vi "AprilTag Target Package Code 1.vi"(0 "Camera List":string[](array[string]), 1 "Instance":i32) -> ()   [LabVIEW 2025]
uses:
  Camera Set Up/Ctrl/White Balance.ctl
  Camera Info.ctl
  State Machine/AprialTag States.ctl
  State Machine/AprialTag Main Cluster.ctl
  <vilib>/vision/Image Controls.llb/IMAQ Image.ctl
  Steam Type.ctl
  Camera Set Up/Event/Event Setup Types.ctl
  <vilib>/Utility/config.llb/Read Key (String).vi
  <vilib>/Utility/config.llb/Write Key (String).vi
  <vilib>/Utility/config.llb/NI_LVConfig.lvlib
  <vilib>/ptbypt/NI_PtbyPt.lvlib
panel:
  in  "Main":T1(tab)
  out "Running":bool
  out "Image":T2(plugin-control)
  out "Camera Name":string="cam0"
  in  "Settings":bool
  out "FPS":dbl format="%#.0f"
  out "Height":i32=360
  out "Width":i32=640
  out "Target Info":dbl[][](array[numeric]) format="%.1f"
  in  "Camera Setting":bool
  in  "Home":bool
  in  "Robot Calibration Cluster":T3={"Camera FOV Vert View Angle (deg)"=75.0, "Camera FOV Hor View Angle (deg)"=90.0, "Distance Correction Factor"=3.952} {"Distance Correction Factor" format="%#_13g"; "Camera FOV Hor View Angle (deg)" format="%#_13g"; "Camera FOV Vert View Angle (deg)" format="%#_13g"}
  in  "decimate":dbl=4.0 format="%#_13g"
  out "Camera Name 2":string="cam0"
  in  "Save":bool
  in  "Timeout":u32
  out "Distance (tag-size units)":dbl
  in  "Gamma":i32(slide)=50 min=0 max=100 scale=0.0..100.0
  in  "Brightness":i32(slide)=50 min=0 max=100 scale=0.0..100.0
  in  "Exposure":dbl(slide)=2.0 min=0.0 max=100.0 step=0.01 scale=0.0..100.0
  in  "Gain":i32(slide)=50 min=0 max=100 scale=0.0..100.0
  in  "Contrast":i32(slide)=50 min=0 max=100 scale=0.0..100.0
  in  "Sharpness":i32(slide)=50 min=0 max=100 scale=0.0..100.0
  in  "VideoMode":u16(ring)=20 items=["640x480 MJPG 60.00fps", "640x480 YUY2 60.00fps", "1280x720 MJPG 60.00fps", "1280x720 YUY2 60.00fps", "1600x1304 MJPG 60.00fps", "1600x1304 YUY2 60.00fps"]
  in  "White Balance":T4=enum."Hold current"
  out "Camera Image":T2(plugin-control)
  in  "Hue":i32(slide)=50 min=0 max=100 scale=0.0..100.0
  in  "Saturation":i32(slide)=50 min=0 max=100 scale=0.0..100.0
  out "Camera Name 3":string="cam0"
  in  "Reset Camera":bool
  in  "Camera Save Settings":bool caption="Save"
  out "Width 2":i32=640 caption="Width"
  out "Height 2":i32=360 caption="Height"
  in  "Home 2":bool caption="Home"
  # "Distance"
  # "Angle"
  # "Tag #"
  # "Yaw"
  # "Pitch"
  # "Roll"
  # "Distance Correction Factor:\nCalibration for the camera. Take three measurements at 24\", 36\", 72\"\n\nCalibration:\ndistance / distance (tag-size units) for each measurement and then average them to get the best correction factor."
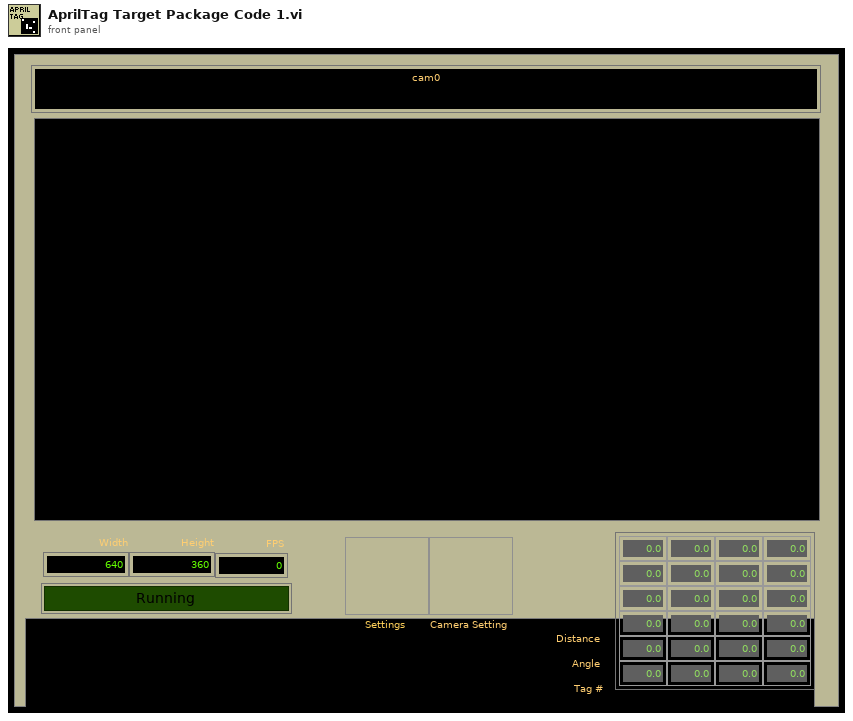
[diagram p1: front panel]
types:
  T1 = enum32{"Main", "Camera Setup", "Camera Settings"}
  T2 = typedef "IMAQ Image.ctl" = refnum<image>
  T3 = typedef "Camera Info.ctl" = cluster{"Camera FOV Vert View Angle (deg)":dbl, "Camera FOV Hor View Angle (deg)":dbl, "Distance Correction Factor":dbl}
  T4 = typedef "White Balance.ctl" = enum16{"Auto", "Fixed indoor", "Fixed outdoor 1", "Fixed outdoor 2", "Fixed fluorescent 1", "Fixed fluorescent 2", "Hold current", "Custom"}
  T5 = typedef "AprialTag Main Cluster.ctl" = cluster{"AprilTage FIFO":T6[], "Camera Name":string, "AprilTag path":path, "Control Ref's":refnum<vi>[], "Main Image":T2, "EDIT Settings":bool, "Camera Number":dbl}
  T6 = typedef "AprialTag States.ctl" = enum16{"Message Dispatcher", "INI", "Open", "Save", "Exit"}
  T7 = typedef "Event Setup Types.ctl" = enum16{"Default", "Camera Loop Started", "GreyScale", "Reset Camera Settings", "Reset Team Number", "Save Data", "Setting Changed", "Update Video Mode", "Video Mode Changed", "Exit"}
  T8 = cluster{"tag ID":i32, "Center":cluster{"X":dbl, "Y":dbl}, "homography matrix":dbl[], "decision margin":dbl, "Hamming Dist":i32, "corner points":cluster{"X":dbl, "Y":dbl}[], "Tag Family":string}[]
  T9 = typedef "AprilTag Target Fields.ctl" = cluster{"diameter points":cluster{"first point":cluster{"x":dbl, "y":dbl}, "projected point":cluster{"x":dbl, "y":dbl}}, "Tag Center":cluster{"X":dbl, "Y":dbl}, "AprilTag Number":i32, "homography matrix":dbl[]}
  T10 = typedef "Image Type" = u32
  T11 = typedef "NI_LVConfig.lvlib/Config Data RefNum.ctl" = refnum<k1>
  T12 = typedef "Steam Type.ctl" = enum8{"Unknown", "Apriltag", "Fuel", "Other"}
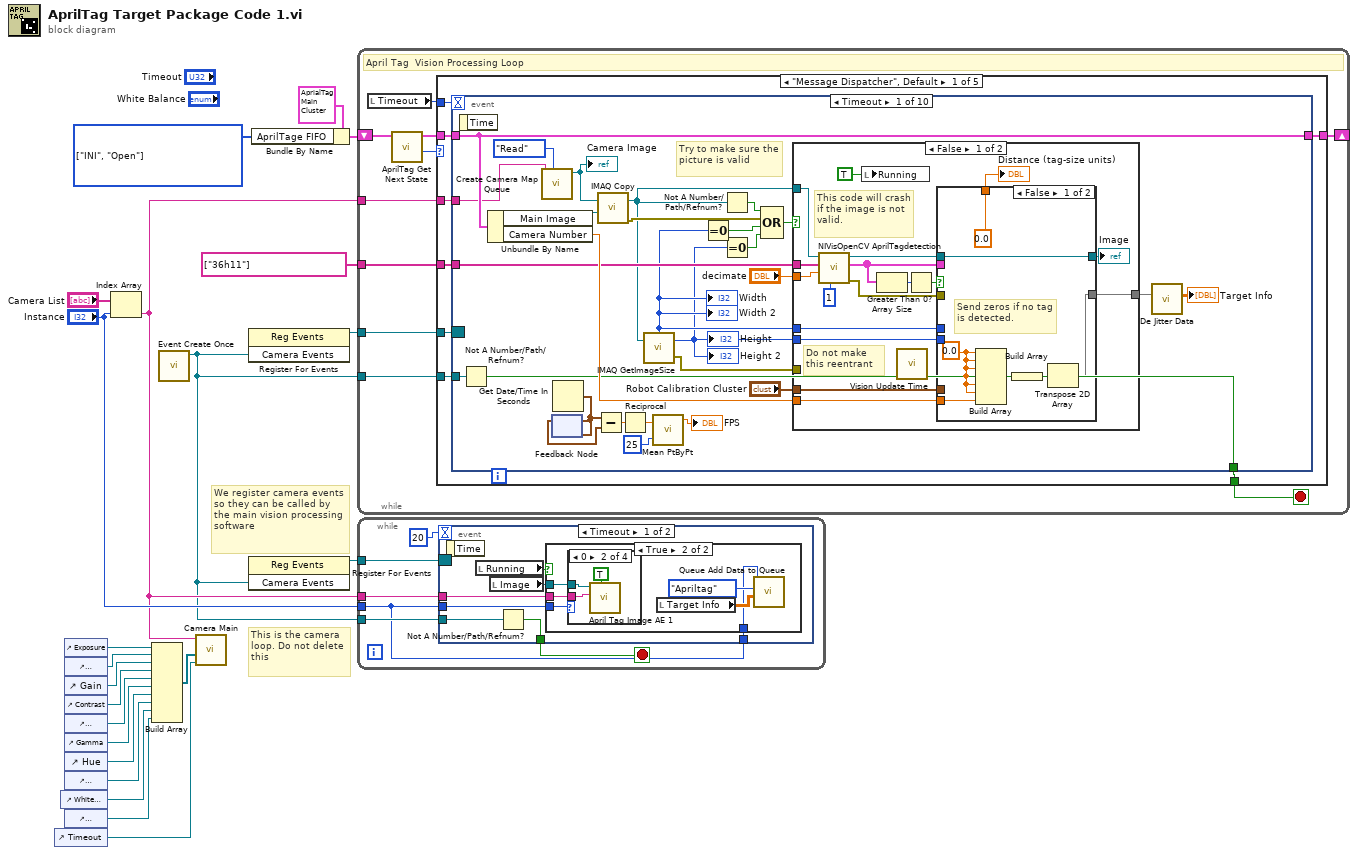
[diagram p0: block diagram]
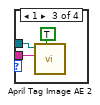
[diagram p4: hidden frame]
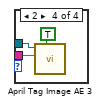
[diagram p5: hidden frame]
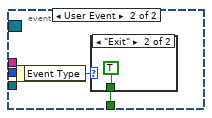
[diagram p6: hidden frame]
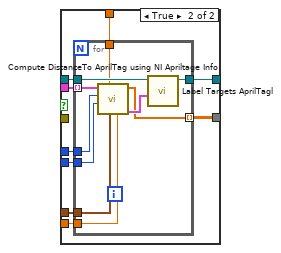
[diagram p8: hidden frame]
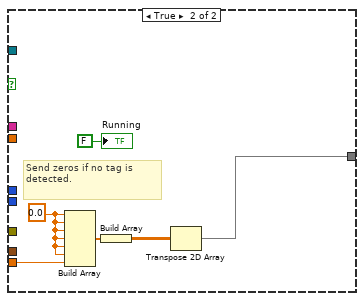
[diagram p9: hidden frame]
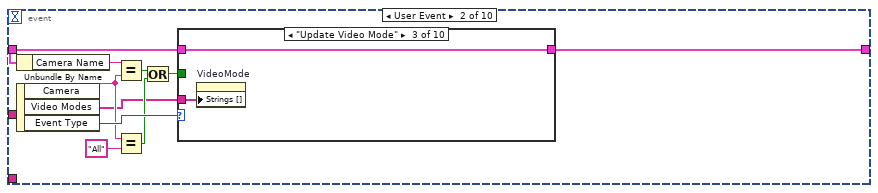
[diagram p10: hidden frame]
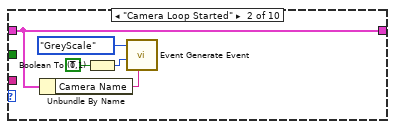
[diagram p12: hidden frame]
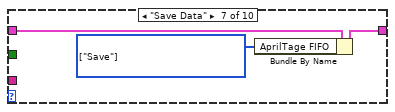
[diagram p16: hidden frame]
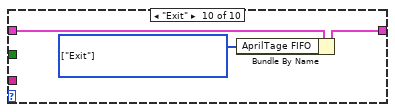
[diagram p19: hidden frame]
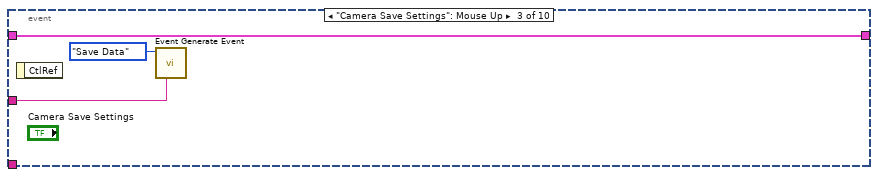
[diagram p20: hidden frame]
diagram:
  w17 = T6[] [enum."INI", enum."Open"] items=["Message Dispatcher", "INI", "Open", "Save", "Exit"] ("AprilTage FIFO")
  # "This is the camera loop. Do not delete this"
  # "We register camera events so they can be called by the main vision processing software"
  n1 = control-ref of="Timeout"() -> (w13:refnum<vi>)
  n2 = control-ref of="White Balance"() -> (w4:refnum<vi>)
  n3 = control-ref of="Exposure"() -> (w5:refnum<vi>)
  n4 = control-ref of="Brightness"() -> (w6:refnum<vi>)
  n5 = control-ref of="Gain"() -> (w7:refnum<vi>)
  n6 = control-ref of="Contrast"() -> (w8:refnum<vi>)
  n7 = control-ref of="Sharpness"() -> (w9:refnum<vi>)
  n8 = control-ref of="Gamma"() -> (w10:refnum<vi>)
  n9 = control-ref of="Hue"() -> (w11:refnum<vi>)
  n10 = control-ref of="Saturation"() -> (w12:refnum<vi>)
  n11 = control-ref of="VideoMode"() -> (w3:refnum<vi>)
  n12 = Index Array(array="Camera List", index="Instance") -> (element=w14:string)
  n13 = Build Array(w5, w6, w7, w8, w9, w10, w11, w12, w4, w3) -> (w2:refnum<vi>[])
  n14 = call "Event Create Once.vi"() -> ("Camera Events"=w1:refnum<user-event>)  [unwired: 10 in, 1 out]
  n15 = call "Camera Main.vi"("Timeout 2"=w13, "Main Open and Save Ctrls Ref"=w2, "Camera"=w14) -> ()  [unwired: 9 in]
  n16 = register-events(w1) -> (reference out=w20:refnum<event-registration>)  [unwired: 2 in, 1 out]
  n17 = register-events(w1) -> (reference out=w15:refnum<event-registration>)  [unwired: 2 in, 1 out]
  n18 = Bundle By Name(cluster=T5 {"AprilTage FIFO"=[], "Camera Name"="", "AprilTag path"=path "", "Control Ref's"=[], "Main Image"=refnum, "EDIT Settings"=FALSE, "Camera Number"=0.0} ("AprilTag Main Cluster out"), "AprilTage FIFO"=w17) -> (w18:T5)
  n19 = while {
    tunnel: w20 -> [w32]
    shift-right: [w28] -> _
    shift-left: w18 -> [w27]
    tunnel: string[] ["36h11"] ("Tag Familys") -> [w26]
    tunnel: w14 -> [w25]
    tunnel: w1 -> [w24]
    stop <- w31 stop-if-true
    # "April Tag  Vision Processing Loop"
    n20 = local read "Timeout"() -> (w23:u32)
    n21 = call "AprilTag Get Next State.vi"("AprilTag Main Cluster in"=w27) -> ("Next State"=w29:T6, "AprilTag Main Cluster out"=w30:T5)  [unwired: 9 in]
    n22 = case shown="\"Message Dispatcher\", Default" w29 {
      tunnel: w32 -> [w40 _ _ _ _]
      tunnel: [w34 _ _ _ TRUE] -> w31
      tunnel: w30 -> [w38 w185 w199 w235 w251]
      tunnel: [w39 w184 w198 w235 w251] -> w28
      tunnel: w23 -> [w37 _ _ _ _]
      tunnel: w26 -> [w36 _ _ _ _]
      tunnel: w25 -> [w33 w175 w187 _ _]
      tunnel: w24 -> [w35 _ _ _ _]
      frame "Message Dispatcher", Default {
        n23 = event shown="[0] Timeout" {
          selector: w40 -> [_ _ _ _ _ _ _ _ _ _]
          dyn-events: _ -> [_ _ _ _ _ _ _ _ _ _]
          timeout: w37 -> [_ _ _ _ _ _ _ _ _ _]
          tunnel: w38 -> [w68 w125 w149 w151 w159 w161 w164 w167 w169 w173]
          tunnel: [w68 w127 w149 w151 w159 w161 w164 w166 w169 w173] -> w39
          tunnel: w36 -> [w64 _ _ _ _ _ _ _ _ _]
          tunnel: w35 -> [w50 _ _ _ _ _ _ _ _ _]
          tunnel: [w49 _ _ _ _ _ _ _ _ _] -> w34
          tunnel: w33 -> [w47 _ w147 _ w157 _ w162 _ _ w170]
          event Timeout {
            # "Try to make sure the picture is valid"
            n24 = event-data() -> ()  [unwired: 1 in, 1 out]
            n25 = Not A Number/Path/Refnum?(number/path/refnum=w50) -> (NaN/Path/Refnum?=w49:bool)
            n26 = Unbundle By Name(w68) -> ("Main Image"=w63:T2, "Camera Number"=w66:dbl)
            n27 = call "Create Camera Map Queue.vi"("Action"=enum16{"Read", "Write"}."Read", "Camera"=w47) -> ("Image out"=w46:T2)  [unwired: 8 in, 1 out]
            "Camera Image" <- w46
            n28 = Get Date/Time In Seconds() -> (seconds since 1Jan1904=w57:timestamp)
            n29 = feedback #1(w57) -> (w58:timestamp)
            n30 = feedback-in #1(w57) -> ()
            n31 = Subtract(x=w57, y=w58) -> (x-y=w55:dbl)
            n32 = call "IMAQ Copy"("Image Dst"=w63, "Image Src"=w46) -> ("error out"=w62:errorcluster, "Image Dst Out"=w59:T2)  [unwired: 4 in]
            n33 = Reciprocal(x=w55) -> (1/x=w56:dbl)
            n34 = call "IMAQ GetImageSize"("Image"=w59) -> ("Y Resolution"=w44:i32, "X Resolution"=w45:i32, "error out"=w41:errorcluster)  [unwired: 3 in]
            "Height" <- w44
            "Width" <- w45
            "Width 2" <- w45
            "Height 2" <- w44
            n35 = call <vilib>:"Mean PtByPt.vi"("x"=w56, "sample length"=25) -> ("mean"=→"FPS":dbl)  [unwired: 2 in, 1 out]
            n36 = Equal To 0?(x=w45) -> (x = 0?=w61:bool)
            n37 = Not A Number/Path/Refnum?(number/path/refnum=w59) -> (NaN/Path/Refnum?=w51:bool)
            n38 = Equal To 0?(x=w44) -> (x = 0?=w60:bool)
            n39 = Compound Arithmetic op=OR(w51, w62, w61, w60) -> (w52:bool)
            n40 = case shown="False" w52 {
              tunnel: w64 -> [w85 _]
              tunnel: "Robot Calibration Cluster" -> [w84 _]
              tunnel: [w71 w112] -> w43
              tunnel: w66 -> [w79 w115]
              tunnel: w59 -> [w76 _]
              tunnel: "decimate" -> [w77 _]
              tunnel: w44 -> [w74 _]
              tunnel: w45 -> [w73 _]
              tunnel: w41 -> [_ _]
              frame False {
                # "Do not make this reentrant"
                # "This code will crash if the image is not valid."
                n41 = call "NIVisOpenCV AprilTagdetection.vi"("threads"=1, "decimate"=w77, "Tag Familys"=w85, "Image Src"=w76) -> ("error out"=w80:errorcluster, "Detected Tags"=w83:T8, "Image Dst Out"=w75:T2)  [unwired: 4 in, 1 out]
                n42 = local write "Running"(TRUE ("Running")) -> ()
                n43 = Array Size(array=w83) -> (size(s)=w82:i32)
                n44 = call "Vision Update Time.vi"() -> ()  [unwired: 12 in]
                n45 = Greater Than 0?(x=w82) -> (x > 0?=w81:bool)
                n46 = case shown="False" w81 {
                  tunnel: w75 -> [w92 w101]
                  tunnel: w83 -> [_ w100]
                  tunnel: [w92 w96] -> w78
                  tunnel: w80 -> [_ _]
                  tunnel: w84 -> [_ w99]
                  tunnel: [w86 w98] -> w71
                  tunnel: w79 -> [w89 w97]
                  tunnel: w74 -> [_ w95]
                  tunnel: w73 -> [_ w94]
                  tunnel: [0.0 ("Distance (tag-size units)") w93] -> w70
                  frame False {
                    w87 = 0.0
                    # "Send zeros if no tag is detected."
                    n47 = Build Array(w87, w87, w87, w87, w87, w87, w89) -> (w91:dbl[])
                    n48 = Build Array(w91) -> (w90:dbl[][])
                    n49 = Transpose 2D Array(2D array=w90) -> (transposed array=w86:dbl[][])
                  }
                  frame True {
                    n50 = for {
                      tunnel: w100 -> [w108] mode=indexing
                      tunnel: w101 -> [w109]
                      tunnel: [w111] -> w96
                      tunnel: w99 -> [w110]
                      tunnel: [w103] -> w98 mode=indexing
                      tunnel: w97 -> [w104]
                      tunnel: w95 -> [w106]
                      tunnel: w94 -> [w107]
                      tunnel: [w102] -> w93
                      n51 = call "Compute DistanceTo AprilTag using NI Apriltage Info.vi"("Camera#"=w104, "Robot Calibration Cluster"=w110, "Y Resolution"=w106, "X Resolution"=w107, "tag info"=w108) -> ("results out"=w105:T9, "Target Info"=w103:dbl[], "Distance (tag-size units)"=w102:dbl)  [unwired: 3 in, 1 out]
                      n52 = call "Label Targets AprilTagl.vi"("results"=w105, "Image in"=w109) -> ("Image out"=w111:T2)  [unwired: 9 in]
                    }
                  }
                }
                "Image" <- w78
                "Distance (tag-size units)" <- w70
              }
              frame True {
                w114 = 0.0
                # "Send zeros if no tag is detected."
                n53 = Build Array(w114, w114, w114, w114, w114, w114, w115) -> (w117:dbl[])
                n54 = Build Array(w117) -> (w116:dbl[][])
                n55 = Transpose 2D Array(2D array=w116) -> (transposed array=w112:dbl[][])
                "Running" <- FALSE ("Running")
              }
            }
            n56 = call "De Jitter Data.vi"("Target Info"=w43) -> ("Filtered Data"=→"Target Info":dbl[][])  [unwired: 10 in]
          }
          event User Event {
            n57 = Unbundle By Name(w125) -> ("Camera Name"=w124:string)
            n58 = event-data() -> ("Camera"=w121:string, "Video Modes"=w118:string[], "Event Type"=w126:T7)  [unwired: 1 in]
            n59 = Equal?(x=w124, y=w121) -> (x = y?=w123:bool)
            n60 = Equal?(x=w121, y="All") -> (x = y?=w119:bool)
            n61 = Or(x=w123, y=w119) -> (x .or. y?=w120:bool)
            n62 = case shown="\"Update Video Mode\"" w126 {
              tunnel: w125 -> [w128 w132 w135 w136 w137 w138 w141 w142 w143 w146]
              tunnel: [w128 w132 w135 w136 w137 w138 w140 w142 w143 w145] -> w127
              tunnel: w120 -> [_ _ _ _ _ _ _ _ _ _]
              tunnel: w118 -> [_ _ w134 _ _ _ _ _ _ _]
              frame "Default" {
              }
              frame "Camera Loop Started" {
                n63 = Unbundle By Name(w132) -> ("Camera Name"=w131:string)
                n64 = Boolean To (0,1)(Boolean=TRUE) -> (0, 1=w129:i16)
                n65 = call "Event Generate Event.vi"("Camera Name"=w131, "Setpoint"=w129, "Event Type"=Event_Setup_Types."GreyScale") -> ()  [unwired: 9 in]
              }
              frame "Update Video Mode" {
                n66 = property on="VideoMode" class="Ring (strict)"("Strings []"=w134) -> ()  [unwired: 2 in, 2 out]
              }
              frame "GreyScale" {
              }
              frame "Reset Camera Settings" {
              }
              frame "Reset Team Number" {
              }
              frame "Save Data" {
                w139 = T6[] [enum."Save"] items=["Message Dispatcher", "INI", "Open", "Save", "Exit"] ("AprilTage FIFO")
                n67 = Bundle By Name(cluster=w141, "AprilTage FIFO"=w139) -> (w140:T5)
              }
              frame "Setting Changed" {
              }
              frame "Video Mode Changed" {
              }
              frame "Exit" {
                w144 = T6[] [enum."Exit"] items=["Message Dispatcher", "INI", "Open", "Save", "Exit"] ("AprilTage FIFO")
                n68 = Bundle By Name(cluster=w146, "AprilTage FIFO"=w144) -> (w145:T5)
              }
            }
          }
          event "Camera Save Settings": Mouse Up {
            n69 = event-data() -> ()  [unwired: 1 in, 1 out]
            n70 = call "Event Generate Event.vi"("Camera Name"=w147, "Event Type"=Event_Setup_Types."Save Data") -> ()  [unwired: 10 in]
          }
          event "Camera Setting": Mouse Up {
            n71 = event-data() -> ()  [unwired: 1 in, 1 out]
            n72 = property on="Main" class="TabCtl (strict)"("Value"=T1."Camera Settings" ("Main")) -> ()  [unwired: 2 in, 2 out]
          }
          event "Gain", "Exposure", "Brightness", "Gamma", "Sharpness", "Contrast", "Saturation", "Hue": Value Change {
            n73 = event-data() -> ("CtlRef"=w156:refnum<vi>)  [unwired: 1 in]
            n74 = property on="Property Node" class="Slide"(reference=w156) -> ("Label.Text"=w155:string, "Value"=w154:variant)  [unwired: 1 in, 2 out]
            n75 = Variant To Data(type=0.0, Variant=w154) -> (data=w152:dbl)  [unwired: 1 in, 1 out]
            n76 = call "Event Generate Event.vi"("Camera Name"=w157, "Setpoint"=w152, "Setting Name"=w155, "Event Type"=Event_Setup_Types."Setting Changed") -> ()  [unwired: 8 in]
          }
          event "Home", "Home 2": Mouse Up {
            n77 = event-data() -> ()  [unwired: 1 in, 1 out]
            n78 = property on="Main" class="TabCtl (strict)"("Value"=T1."Main" ("Main")) -> ()  [unwired: 2 in, 2 out]
          }
          event "Reset Camera": Mouse Up {
            n79 = event-data() -> ()  [unwired: 1 in, 1 out]
            n80 = call "Event Generate Event.vi"("Camera Name"=w162, "Event Type"=Event_Setup_Types."Reset Camera Settings") -> ()  [unwired: 10 in]
          }
          event "Save": Mouse Up {
            w165 = T6[] [enum."Save"] items=["Message Dispatcher", "INI", "Open", "Save", "Exit"] ("AprilTage FIFO")
            n81 = event-data() -> ()  [unwired: 1 in, 1 out]
            n82 = Bundle By Name(cluster=w167, "AprilTage FIFO"=w165) -> (w166:T5)
          }
          event "Settings": Mouse Up {
            n83 = event-data() -> ()  [unwired: 1 in, 1 out]
            n84 = property on="Main" class="TabCtl (strict)"("Value"=T1."Camera Setup" ("Main")) -> ()  [unwired: 2 in, 2 out]
          }
          event "VideoMode": Value Change {
            n85 = event-data() -> ("NewVal"=w171:u16)  [unwired: 1 in]
            n86 = call "Event Generate Event.vi"("Camera Name"=w170, "Setpoint"=w171, "Event Type"=Event_Setup_Types."Video Mode Changed") -> ()  [unwired: 9 in]
          }
        }
      }
      frame "INI" {
        w183 = T10 0 items=["Grayscale (U8)", "Grayscale (I16)", "Grayscale (SGL)", "Complex (CSG)", "RGB (U32)", "HSL (U32)", "RGB (U64)", "Grayscale (U16)"] ("Image Type")
        n87 = Match Pattern(string=w175, regular expression="[1-9]") -> (match substring=w177:string)  [unwired: 1 in, 3 out]
        n88 = Concatenate Strings(w175, "AprilTag Main" ("string")) -> (w182:string)
        n89 = Fract/Exp String To Number(string=w177) -> (number=w176:dbl)  [unwired: 3 in, 1 out]
        n90 = call "IMAQ Create"("Image Name"=w182, "Image Type"=w183) -> ("New Image"=w180:T2)  [unwired: 2 in, 2 out]
        n91 = Bundle By Name(cluster=w185, "Camera Name"=w175, "Main Image"=w180, "EDIT Settings"=FALSE, "Camera Number"=w176) -> (w184:T5)
        n92 = property on="Main" class="TabCtl (strict)"("Value"=T1."Main" ("Main")) -> ()  [unwired: 2 in, 2 out]
        "Camera Name" <- w175
        "Camera Name 3" <- w175
        "Camera Name 2" <- w175
      }
      frame "Open" {
        n93 = call "Attached Camera Info AE.vi"("InterfaceName"=w187) -> ("Serial Number"=w186:string)  [unwired: 10 in]
        n94 = call <vilib>:"Application Directory.vi"() -> ("Application Directory"=w202:path)
        n95 = Concatenate Strings(w186, ".ini" ("name or relative path")) -> (w210:string)
        n96 = Build Path(base path=w202, name or relative path="Config") -> (appended path=w200:path)
        n97 = Build Path(base path=w200, name or relative path=w210) -> (appended path=w194:path)
        n98 = call <vilib>:"Check if File or Folder Exists.vi"("error in (no error)"=errorcluster {"status"=FALSE, "code"=0, "source"=""}, "path"=w194) -> ("error out"=w190:errorcluster, "file or folder exists?"=w192:bool, "dup path"=w193:path)  [unwired: 7 in]
        n99 = control-ref of="Robot Calibration Cluster"() -> (w205:refnum<vi>)
        n100 = control-ref of="decimate"() -> (w188:refnum<vi>)
        n101 = case shown="True" w192 {
          tunnel: [w213 w214] -> w203
          tunnel: w193 -> [w212 w215]
          tunnel: [w212 w215] -> w191
          tunnel: w190 -> [w211 w214]
          frame False {
            n102 = call <vilib>:"Create File and Containing Folders.vi"("error in (no error)"=w211, "file path"=w212) -> ("error out"=w213:errorcluster)  [unwired: 8 in, 1 out]
          }
          frame True {
          }
        }
        n103 = Build Array(w205, w188) -> (w197:refnum<vi>[])
        n104 = call <vilib>:"Open Config Data.vi"("error in (no error)"=w203, "configuration file path"=w191) -> ("error out"=w206:errorcluster, "refnum"=w209:T11)  [unwired: 7 in, 1 out]
        n105 = for {
          tunnel: "Info" ("Camera Name") -> [w228]
          tunnel: w197 -> [w226] mode=indexing
          shift-right: [w230] -> w208
          shift-left: w209 -> [w231]
          shift-right: [w229] -> w207
          shift-left: w206 -> [w227]
          tunnel: [w221] -> _ mode=indexing
          tunnel: errorcluster {"status"=FALSE, "code"=0, "source"=""} ("error out") -> [w220]
          tunnel: [w216] -> _ mode=indexing
          n106 = property on="Property Node" class="Ctl"(reference=w226, error in=w220) -> (reference out=w224:refnum<vi>, error out=w222:errorcluster, "Label.Text"=w225:string, "Value"=w218:variant)
          n107 = Variant To Flattened String(Variant=w218) -> (1:w217:i16[])  [unwired: 1 out]
          n108 = call-poly <vilib>:"Read Key.vi"("section"=w228, "error in (no error)"=w227, "key"=w225, "refnum"=w231) -> ("error out"=w229:errorcluster, "value"=w223:string, "refnum out"=w230:T11)  [unwired: 4 in, 1 out]
          n109 = Flattened String To Variant(6:w223, 7:w217) -> (0:w216:errorcluster, 3:w219:variant)  [unwired: 1 in]
          n110 = property on="Property Node" class="Ctl"(reference=w224, error in=w222, "Value"=w219) -> (error out=w221:errorcluster)  [unwired: 1 out]
        }
        n111 = call <vilib>:"Close Config Data.vi"("error in (no error)"=w207, "refnum"=w208) -> ()  [unwired: 8 in, 2 out]
        n112 = Bundle By Name(cluster=w199, "Control Ref's"=w197, "AprilTag path"=w191) -> (w198:T5)
      }
      frame "Save" {
        n113 = Unbundle By Name(w235) -> ("Control Ref's"=w233:refnum<vi>[], "AprilTag path"=w234:path)
        n114 = call <vilib>:"Open Config Data.vi"("configuration file path"=w234) -> ("error out"=w236:errorcluster, "refnum"=w239:T11)  [unwired: 8 in, 1 out]
        n115 = for {
          tunnel: "Info" ("Camera Name") -> [w245]
          shift-right: [w248] -> w238
          shift-left: w239 -> [w249]
          shift-right: [w247] -> w237
          shift-left: w236 -> [w246]
          tunnel: w233 -> [w240] mode=indexing
          n116 = property on="Property Node" class="Ctl"(reference=w240, error in=w246) -> (error out=w242:errorcluster, "Label.Text"=w244:string, "Value"=w243:variant)  [unwired: 1 out]
          n117 = Variant To Flattened String(Variant=w243) -> (data string=w241:string)  [unwired: 1 out]
          n118 = call-poly <vilib>:"Write Key.vi"("section"=w245, "error in (no error)"=w242, "value"=w241, "key"=w244, "refnum"=w249) -> ("error out"=w247:errorcluster, "refnum out"=w248:T11)  [unwired: 4 in, 1 out]
        }
        n119 = call <vilib>:"Close Config Data.vi"("error in (no error)"=w237, "refnum"=w238) -> ()  [unwired: 8 in, 2 out]
      }
      frame "Exit" {
        n120 = Unbundle By Name(w251) -> ("Main Image"=w250:T2)
        n121 = call "IMAQ Dispose"("Image"=w250) -> ()  [unwired: 5 in, 1 out]
      }
    }
  }
  n122 = while {
    tunnel: w15 -> [w258]
    tunnel: "Instance" -> [w253]
    tunnel: w14 -> [w256]
    tunnel: w1 -> [w255]
    stop <- w257 stop-if-true
    n123 = event shown="[0] Timeout" {
      selector: w258 -> [_ _]
      dyn-events: _ -> [_ _]
      timeout: 20 -> [_ _]
      tunnel: [w260 w281] -> w257
      tunnel: w253 -> [w264 _]
      tunnel: w256 -> [w262 _]
      tunnel: w255 -> [w261 _]
      tunnel: w253 -> [w259 _]
      event Timeout {
        n124 = event-data() -> ()  [unwired: 1 in, 1 out]
        n125 = local read "Running"() -> (w263:bool)
        n126 = local read "Image"() -> (w265:T2)
        n127 = Not A Number/Path/Refnum?(number/path/refnum=w261) -> (NaN/Path/Refnum?=w260:bool)
        n128 = case shown="True" w263 {
          tunnel: w265 -> [_ w271]
          tunnel: w264 -> [_ w270]
          tunnel: w262 -> [_ w268]
          tunnel: w259 -> [_ w266]
          frame False {
          }
          frame True {
            n129 = case shown="0" w270 {
              tunnel: w271 -> [_ w273 w277 w280]
              tunnel: w268 -> [_ w272 w276 w279]
              frame Default {
              }
              frame 0 {
                n130 = call "April Tag Image AE 1.vi"("Update"=TRUE, "Camera Name"=w272, "Apriltag Image in"=w273) -> ()  [unwired: 8 in, 1 out]
              }
              frame 1 {
                n131 = call "April Tag Image AE 2.vi"("Update"=TRUE, "Camera Name"=w276, "Apriltag Image in"=w277) -> ()  [unwired: 8 in, 1 out]
              }
              frame 2 {
                n132 = call "April Tag Image AE 3.vi"("Update"=TRUE, "Camera Name"=w279, "Apriltag Image in"=w280) -> ()  [unwired: 8 in, 1 out]
              }
            }
            n133 = local read "Target Info"() -> (w269:dbl[][])
            n134 = call "Queue Add Data to Queue.vi"("Target Info in"=w269, "Stream Type"=Steam_Type."Apriltag", "Camera Index"=w266) -> ()  [unwired: 9 in]
          }
        }
      }
      event User Event {
        n135 = event-data() -> ("Event Type"=w282:T7)  [unwired: 1 in]
        n136 = case shown="\"Exit\"" w282 {
          tunnel: [_ TRUE] -> w281
          frame Default {
          }
          frame "Exit" {
          }
        }
      }
    }
  }
